vi "Push_Data_Client.vi"(4 "Archive File?":bool[](array[boolean]), 5 "Running on Server?":bool, 6 "application reference":refnum<vi>, 7 "error in (no error)":errorcluster, 8 "File to transfer":path[](array[path]), 9 "Relative Path":path=path "/Lacie_20/test", 10 "Local Path":path) -> (0 "error out":errorcluster)   [LabVIEW 2011]
uses:
  Anemometry/Anemometry Sub Vis/Globals/Constants_global.vi
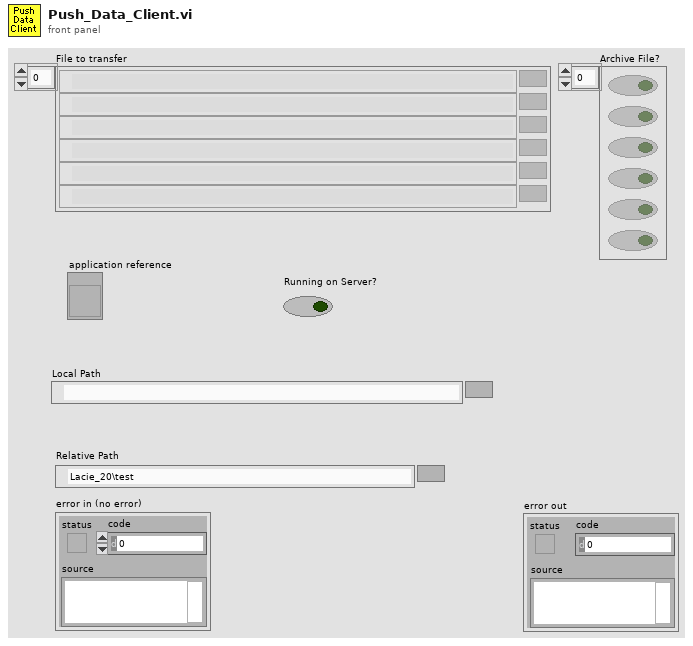
[diagram p1: front panel]
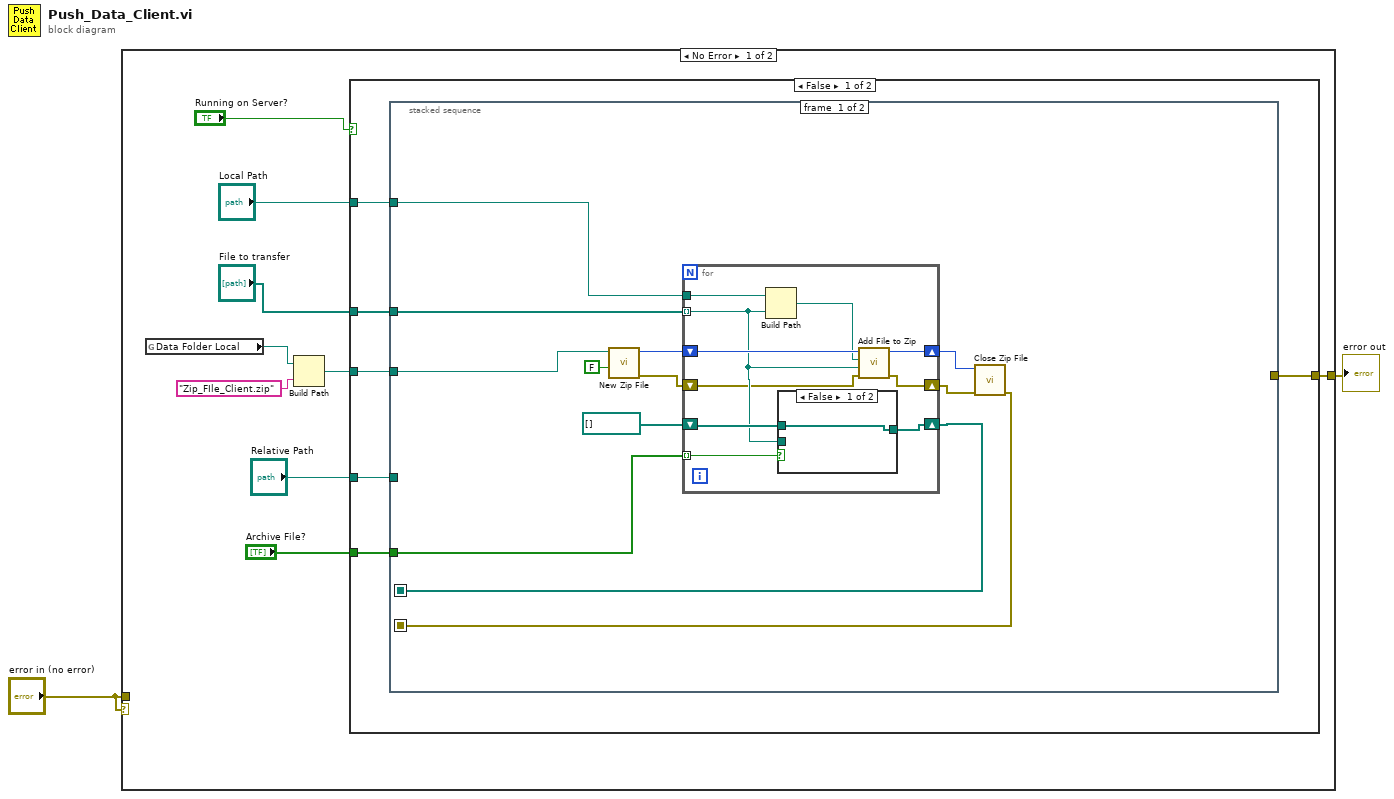
[diagram p0: block diagram]
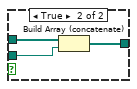
[diagram p2: hidden frame]
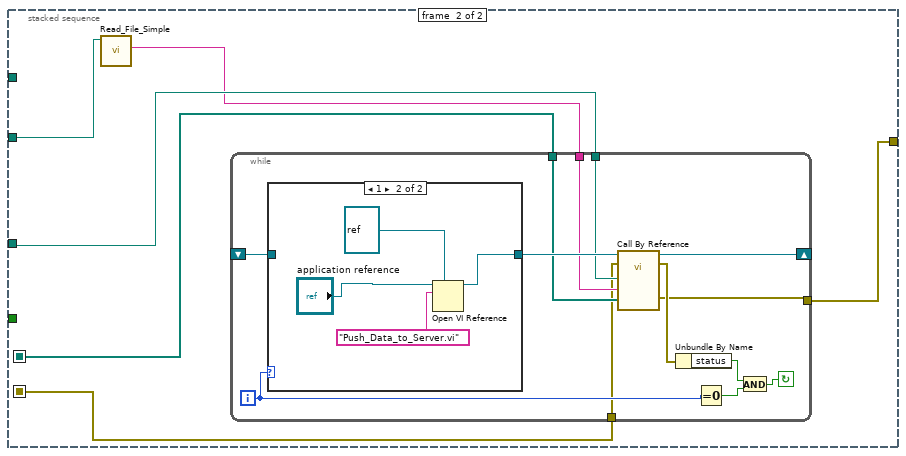
[diagram p3: hidden frame]
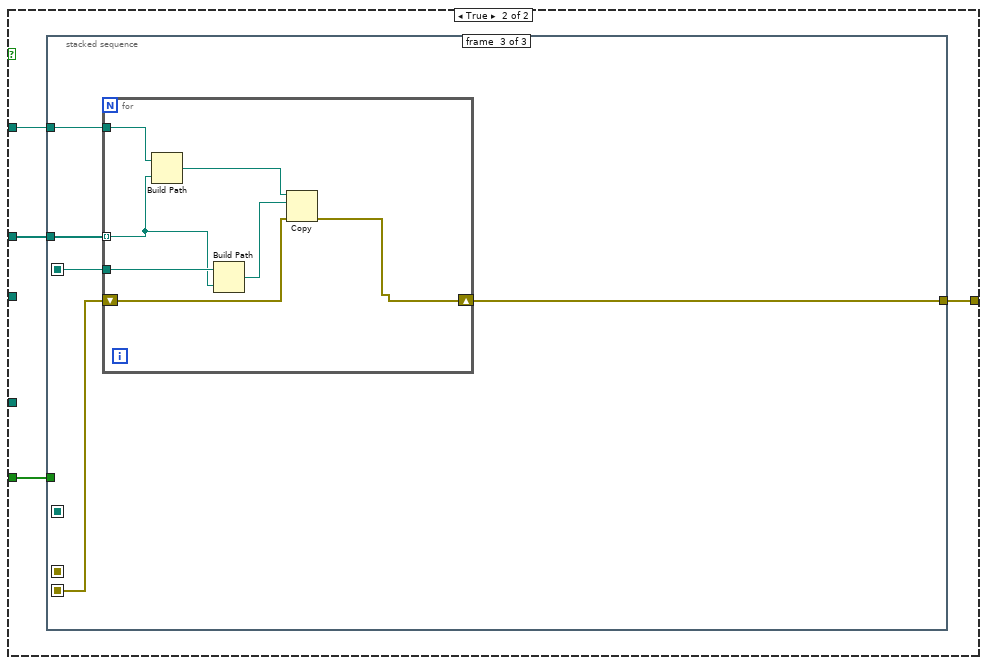
[diagram p5: hidden frame]
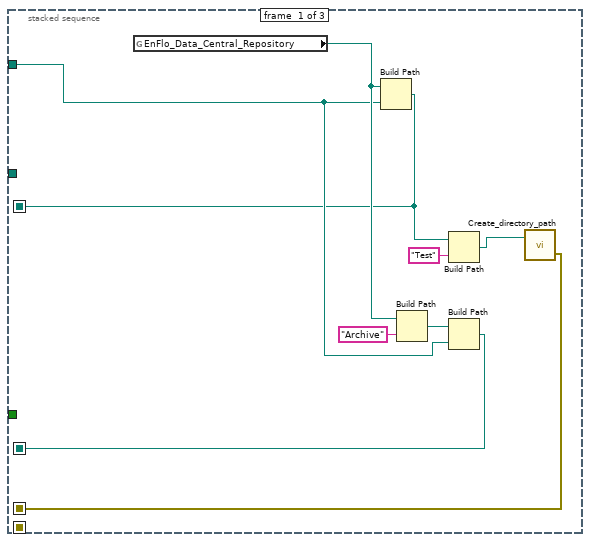
[diagram p6: hidden frame]
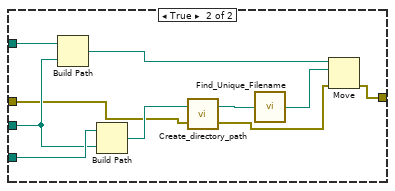
[diagram p8: hidden frame]
diagram:
  n1 = case shown="No Error" "error in (no error)" {
    tunnel: [w3 w116] -> w2
    tunnel: "error in (no error)" -> [_ w116]
    frame No Error {
      n2 = global read "Constants_global.vi" "Data Folder Local"() -> (w11:path)
      n3 = Build Path(base path=w11, name or relative path="Zip_FIle_Client.zip") -> (appended path=w9:path)
      n4 = case shown="False" "Running on Server?" {
        tunnel: w9 -> [w17 _]
        tunnel: "Relative Path" -> [w16 _]
        tunnel: "Local Path" -> [w15 w71]
        tunnel: "File to transfer" -> [w14 w70]
        tunnel: "Archive File?" -> [w13 w69]
        tunnel: [w12 w68] -> w3
        frame False {
          n5 = stacked-sequence {
            seq-local: [w24 _] -> [_ w46]
            seq-local: [w18 _] -> [_ w45]
            tunnel: w17 -> [w26 w49]
            tunnel: w16 -> [_ w48]
            tunnel: w15 -> [w23 _]
            tunnel: w14 -> [w22 _]
            tunnel: w13 -> [w21 _]
            tunnel: [_ w44] -> w12
            frame #0 {
              n6 = call <vilib>:"New Zip File.vi"("confirm overwrite? (F)"=FALSE, "target"=w26) -> ("error out"=w20:errorcluster, "zip file out"=w28:i64)  [unwired: 3 in, 1 out]
              n7 = for {
                shift-right: [w38] -> w29
                shift-left: w28 -> [w39]
                tunnel: w23 -> [w37]
                tunnel: w22 -> [w32] mode=indexing
                tunnel: w21 -> [w35] mode=indexing
                shift-right: [w33] -> w24
                shift-left: path[] [] -> [w34]
                shift-right: [w30] -> w19
                shift-left: w20 -> [w31]
                n8 = Build Path(base path=w37, name or relative path=w32) -> (appended path=w36:path)
                n9 = case shown="False" w35 {
                  tunnel: w34 -> [w40 w43]
                  tunnel: [w40 w42] -> w33
                  tunnel: w32 -> [_ w41]
                  frame False {
                  }
                  frame True {
                    n10 = Build Array (concatenate)(w43, w41) -> (w42:path[])
                  }
                }
                n11 = call <vilib>:"Add File to Zip.vi"("error in (no error)"=w31, "destination path in zip"=w32, "source file path"=w36, "zip file in"=w39) -> ("error out"=w30:errorcluster, "zip file out"=w38:i64)  [unwired: 6 in]
              }
              n12 = call <vilib>:"Close Zip File.vi"("error in (no error)"=w19, "zip file in"=w29) -> ("error out"=w18:errorcluster)  [unwired: 5 in]
            }
            frame #1 {
              n13 = call "Read_File_Simple.vi"("Filename"=w49) -> ("string"=w47:string)  [unwired: 4 in, 5 out]
              n14 = while {
                shift-right: [w60] -> _
                shift-left: _ -> [w62]
                tunnel: w48 -> [w55]
                tunnel: w47 -> [w54]
                tunnel: w46 -> [w53]
                tunnel: w45 -> [w52]
                tunnel: [w50] -> w44
                i -> [w59]
                stop <- w56 continue-if-true
                n15 = case shown="1" w59 {
                  tunnel: w62 -> [w63 _]
                  tunnel: [w63 w67] -> w61
                  frame 0, Default {
                  }
                  frame 1 {
                    n16 = Open VI Reference(type specifier VI Refnum (for type only)=refnum<vi> refnum ("Push Data Server"), application reference (local)="application reference", vi path="Push_Data_to_Server.vi") -> (vi reference=w67:refnum<vi>)  [unwired: 1 in, 3 out]
                  }
                }
                n17 = call-by-ref "?"(reference=w61, error in=w52, "File to Archive"=w53, "Zip String"=w54, "Relative Path"=w55) -> (reference out=w60:refnum<vi>, error out=w51:errorcluster, "error out"=w50:errorcluster)  [unwired: 1 in]
                n18 = Unbundle By Name(w51) -> ("status"=w57:bool)
                n19 = Equal To 0?(x=w59) -> (x = 0?=w58:bool)
                n20 = And(x=w57, y=w58) -> (x .and. y?=w56:bool)
              }
            }
          }
        }
        frame True {
          n21 = stacked-sequence {
            seq-local: [w74 _ _] -> [_ w86 w106]
            seq-local: [w73 _ _] -> [_ w84 _]
            seq-local: [w72 _ _] -> [_ w82 _]
            seq-local: [_ w81 _] -> [_ _ w105]
            tunnel: w71 -> [w75 _ w108]
            tunnel: w70 -> [_ w85 w107]
            tunnel: w69 -> [_ w83 _]
            tunnel: [_ _ w104] -> w68
            frame #0 {
              n22 = global read "Constants_global.vi" "EnFlo_Data_Central_Repository"() -> (w80:path)
              n23 = Build Path(base path=w80, name or relative path=w75) -> (appended path=w74:path)
              n24 = Build Path(base path=w80, name or relative path="Archive") -> (appended path=w79:path)
              n25 = Build Path(base path=w74, name or relative path="Test") -> (appended path=w76:path)
              n26 = Build Path(base path=w79, name or relative path=w75) -> (appended path=w73:path)
              n27 = call "Create_directory_path.vi"("Path name"=w76) -> ("error out"=w72:errorcluster)  [unwired: 1 in, 1 out]
            }
            frame #1 {
              n28 = for {
                tunnel: w86 -> [w92]
                tunnel: w85 -> [w90] mode=indexing
                tunnel: w84 -> [w91]
                tunnel: w83 -> [w89] mode=indexing
                shift-right: [w87] -> w81
                shift-left: w82 -> [w88]
                n29 = case shown="False" w89 {
                  tunnel: w92 -> [_ w103]
                  tunnel: w91 -> [_ w101]
                  tunnel: w90 -> [_ w100]
                  tunnel: w88 -> [w93 w96]
                  tunnel: [w93 w94] -> w87
                  frame False {
                  }
                  frame True {
                    n30 = Build Path(base path=w103, name or relative path=w100) -> (appended path=w102:path)
                    n31 = Build Path(base path=w101, name or relative path=w100) -> (appended path=w98:path)
                    n32 = call "Create_directory_path.vi"("error in (no error)"=w96, "Path name"=w98) -> ("error out"=w95:errorcluster, "Path name Out"=w97:path)
                    n33 = call "Find_Unique_Filename.vi"("Path In"=w97) -> ("Unique Path Out"=w99:path)  [unwired: 2 in]
                    n34 = Move(source path=w102, error in=w95, 10:w99) -> (error out=w94:errorcluster)  [unwired: 2 in, 2 out]
                  }
                }
              }
            }
            frame #2 {
              n35 = for {
                tunnel: w108 -> [w115]
                tunnel: w107 -> [w113] mode=indexing
                tunnel: w106 -> [w114]
                shift-right: [w109] -> w104
                shift-left: w105 -> [w110]
                n36 = Build Path(base path=w115, name or relative path=w113) -> (appended path=w111:path)
                n37 = Build Path(base path=w114, name or relative path=w113) -> (appended path=w112:path)
                n38 = Copy(8:w110, 10:w112, 11:w111) -> (0:w109:errorcluster)  [unwired: 2 in, 2 out]
              }
            }
          }
        }
      }
    }
    frame Error {
    }
  }
  "error out" <- w2
